vi "Culab Read RF Bin without indicator and warmup.vi"(11 "file path":path=path "E:/TEMP.BIN") -> (3 "exec time":dbl)   [LabVIEW 2020]
uses:
  <vilib>/Ngene/CuLab - GPU Accelerated Toolkit/Toolkit/Low_Level/Tensor_Classes/T_Children/T2D/Controls/T2D_Dims.ctl
  <vilib>/Ngene/CuLab - GPU Accelerated Toolkit/Toolkit/API/Array/Controls/Array_Major.ctl
  <vilib>/Ngene/CuLab - GPU Accelerated Toolkit/Toolkit/Low_Level/Tensor_Classes/T_Children/T1D/T1D_Children/T1D_I16/T1D_I16.lvclass
  C:/Program Files/National Instruments/LabVIEW 2020/vi.lib/Ngene/CuLab - GPU Accelerated Toolkit/Toolkit/Low_Level/Tensor_Classes/T_Children/T1D/T1D.lvclass
  <vilib>/Ngene/CuLab - GPU Accelerated Toolkit/Toolkit/Low_Level/Tensor_Classes/T_Children/T1D/T1D_Children/T1D_CSG/T1D_CSG.lvclass
  <vilib>/Ngene/CuLab - GPU Accelerated Toolkit/Toolkit/Low_Level/Tensor_Classes/T_Children/T1D/T1D_Children/T1D_SGL/Create.vi
  <vilib>/Ngene/CuLab - GPU Accelerated Toolkit/Toolkit/Low_Level/Tensor_Classes/T_Children/T1D/T1D_Children/T1D_I16/Create.vi
  <vilib>/Ngene/CuLab - GPU Accelerated Toolkit/Toolkit/Low_Level/Tensor_Classes/T_Children/T1D/T1D_Children/T1D_CSG/Create.vi
  <vilib>/Ngene/CuLab - GPU Accelerated Toolkit/Toolkit/Low_Level/Tensor_Classes/T_Children/T1D/T1D_Children/T1D_I16/Push.vi
  <vilib>/Ngene/CuLab - GPU Accelerated Toolkit/Toolkit/API/Numeric/Conversion  (API)/SGL/CU_To_SGL_T1D.vi
  <vilib>/Ngene/CuLab - GPU Accelerated Toolkit/Toolkit/API/Numeric/Divide/T1D/CU_DivideC_T1D_SGL.vi
  <vilib>/Ngene/CuLab - GPU Accelerated Toolkit/Toolkit/API/Array/Reshape Array  (API)/CU_Reshape_to_T2D/T1D/CU_Reshape_to_T2D_(T1D_SGL).vi
  <vilib>/Ngene/CuLab - GPU Accelerated Toolkit/Toolkit/API/Array/Index Array Subset/T2D/CU_Index_Array_Subset_T2D_SGL.vi
  <vilib>/Ngene/CuLab - GPU Accelerated Toolkit/Toolkit/API/Numeric/Complex  (API)/Re Im To Complex/T1D/CU_Re_Im_To_Complex_T1D_SGL.vi
  <vilib>/Ngene/CuLab - GPU Accelerated Toolkit/Toolkit/API/Signal Processing/Transforms/CU_FFT/T1D/CU_FFT_T1D_C2C.vi
  <vilib>/Ngene/CuLab - GPU Accelerated Toolkit/Toolkit/API/Array/Array Size/CU_Array_Size_T1D.vi
  <vilib>/Ngene/CuLab - GPU Accelerated Toolkit/Toolkit/API/Numeric/Divide/T1D/CU_DivideC_T1D_CSG.vi
  <vilib>/Ngene/CuLab - GPU Accelerated Toolkit/Toolkit/API/Numeric/Complex  (API)/Complex to Polar/T1D/CU_Complex_to_Polar_T1D_CSG.vi
  <vilib>/Ngene/CuLab - GPU Accelerated Toolkit/Toolkit/API/Elementary/Exponential/Logarithm Base 10/T1D/CU_Logarithm_Base_10_T1D_SGL.vi
  <vilib>/Ngene/CuLab - GPU Accelerated Toolkit/Toolkit/API/Numeric/Multiply/T1D/CU_MultiplyC_T1D_SGL.vi
  <vilib>/Ngene/CuLab - GPU Accelerated Toolkit/Toolkit/API/Numeric/Add/T1D/CU_AddC_T1D_SGL.vi
  <vilib>/Ngene/CuLab - GPU Accelerated Toolkit/Toolkit/Low_Level/Tensor_Classes/T_Children/T1D/T1D_Children/T1D_SGL/Pull.vi
  <vilib>/Ngene/CuLab - GPU Accelerated Toolkit/Toolkit/CuLab.lvlib
  <vilib>/Ngene/CuLab - GPU Accelerated Toolkit/Toolkit/Low_Level/Tensor_Classes/T_Children/T1D/T1D_Children/T1D_SGL/T1D_SGL.lvclass
  <vilib>/Ngene/CuLab - GPU Accelerated Toolkit/Toolkit/Low_Level/Tensor_Classes/T_Children/T2D/T2D_Children/T2D_CDB/T2D_CDB.lvclass
  C:/Program Files/National Instruments/LabVIEW 2020/vi.lib/Ngene/CuLab - GPU Accelerated Toolkit/Toolkit/Low_Level/Tensor_Classes/Tensor.lvclass
  C:/Program Files/National Instruments/LabVIEW 2020/vi.lib/Ngene/CuLab - GPU Accelerated Toolkit/Toolkit/Low_Level/Tensor_Classes/T_Children/T1D/T1D_Children/T1D_I16/T1D_I16.lvclass
  C:/Program Files/National Instruments/LabVIEW 2020/vi.lib/Ngene/CuLab - GPU Accelerated Toolkit/Toolkit/Low_Level/Tensor_Classes/T_Children/T1D/T1D_Children/T1D_CSG/T1D_CSG.lvclass
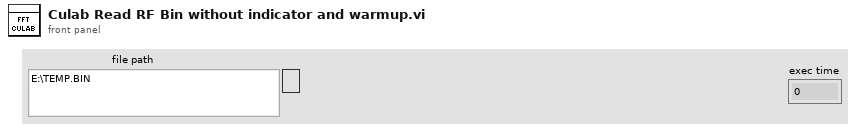
[diagram p1: front panel]
types:
  T1 = enum16{"open", "replace", "create", "open or create", "replace or create", "replace or create with confirmation"}
  T2 = typedef "CuLab.lvlib/T2D_Dims.ctl" = cluster{"H":i32, "W":i32}
  T3 = enum16{"big-endian, network order", "native, host order", "little-endian"}
  T4 = typedef "CuLab.lvlib/Array_Major.ctl" = enum16{"Row", "Column"}
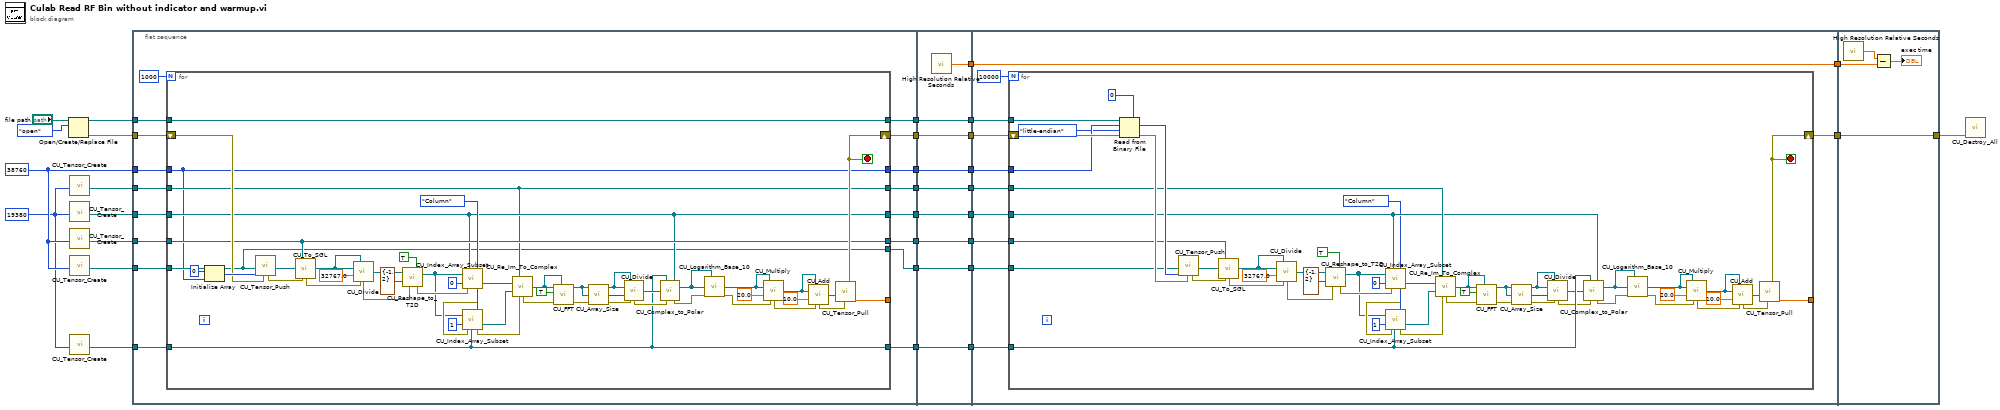
[diagram p0: block diagram]
diagram:
  w21 = 19380 ("count (1)")
  w24 = 38760 ("count (1)")
  n1 = Open/Create/Replace File(file path (use dialog)="file path", operation (0:open)=T1."open") -> (refnum out=w29:refnum<file>, error out=w9:errorcluster)  [unwired: 4 in, 1 out]
  n2 = call-poly <vilib>:"CU_Tensor_Create.vi"("Length"=w21) -> ("T1D_CSG out"=w26:refnum<class "T1D_CSG.lvclass">)  [unwired: 9 in, 1 out]
  n3 = call-poly <vilib>:"CU_Tensor_Create.vi"("Length"=w21) -> ("T1D_SGL out"=w25:refnum<class "T1D_SGL.lvclass">)  [unwired: 9 in, 1 out]
  n4 = call-poly <vilib>:"CU_Tensor_Create.vi"("Length"=w24) -> ("T1D_SGL out"=w27:refnum<class "T1D_SGL.lvclass">)  [unwired: 9 in, 1 out]
  n5 = call-poly <vilib>:"CU_Tensor_Create.vi"("Length"=w24) -> ("T1D_I16 out"=w28:refnum<class "T1D_I16.lvclass">)  [unwired: 9 in, 1 out]
  n6 = call-poly <vilib>:"CU_Tensor_Create.vi"("Length"=w21) -> ("T1D_SGL out"=w23:refnum<class "T1D_SGL.lvclass">)  [unwired: 9 in, 1 out]
  n7 = flat-sequence {
    tunnel: w9 -> [w47]
    tunnel: w23 -> [w43]
    tunnel: w24 -> [w45]
    tunnel: w25 -> [w41]
    tunnel: w26 -> [w40]
    tunnel: w27 -> [w42]
    tunnel: w28 -> [w44]
    tunnel: w29 -> [w46]
    tunnel: [w36] -> w8
    tunnel: [w39] -> w7
    tunnel: [w38] -> w6
    tunnel: [w37] -> w5
    tunnel: [w35] -> w4
    tunnel: [w34] -> w3
    tunnel: [w33] -> w2
    tunnel: [w32] -> w1
    tunnel: [w105] -> w20
    tunnel: [w104] -> w19
    tunnel: [w103] -> w18
    tunnel: [w102] -> w17
    tunnel: [w101] -> w16
    tunnel: [w100] -> w15
    tunnel: [w99] -> w14
    tunnel: [w98] -> w12
    tunnel: [w97] -> w10
    tunnel: w8 -> [w104]
    tunnel: w7 -> [w103]
    tunnel: w6 -> [w101]
    tunnel: w5 -> [w102]
    tunnel: w4 -> [w99]
    tunnel: w3 -> [w97]
    tunnel: w2 -> [w105]
    tunnel: w1 -> [w100]
    tunnel: w20 -> [w115]
    tunnel: w19 -> [w114]
    tunnel: w18 -> [w113]
    tunnel: w17 -> [w112]
    tunnel: w16 -> [w111]
    tunnel: w15 -> [w110]
    tunnel: w14 -> [w109]
    tunnel: [w108] -> w13
    tunnel: w12 -> [w107]
    tunnel: [w107] -> w11
    tunnel: w10 -> [w106]
    tunnel: [w170] -> w22
    tunnel: w13 -> [w170]
    tunnel: w11 -> [w168]
    frame #0 {
      n8 = for {
        N: 1000 -> [_]
        shift-right: [w94] -> w34
        shift-left: w47 -> [w56]
        tunnel: w46 -> [w50]
        tunnel: w44 -> [w52]
        tunnel: w45 -> [w49]
        tunnel: w42 -> [w55]
        tunnel: w40 -> [w53]
        tunnel: w41 -> [w54]
        tunnel: w43 -> [w51]
        tunnel: [w59] -> _
        tunnel: [w55] -> w39
        tunnel: [w54] -> w38
        tunnel: [w53] -> w37
        tunnel: [w52] -> w36
        tunnel: [w51] -> w35
        tunnel: [w50] -> w33
        tunnel: [w49] -> w32
        stop <- w94 stop-if-true
        w87 = Array_Major."Column" ("Row/Column Selector")
        n9 = Initialize Array(i16 0 ("element"), w49) -> (w57:i16[])
        n10 = call-poly <vilib>:"CU_Tensor_Push.vi"("error in (no error)"=w56, "T1D_I16_Data"=w57, "T1D_I16 in"=w52) -> ("T1D_I16 out"=w82:refnum<class "T1D_I16.lvclass">, "error out"=w74:errorcluster)  [unwired: 7 in]
        n11 = call-poly <vilib>:"CU_To_SGL.vi"("Dest in"=w55, "Tensor in"=w82, "error in (no error)"=w74) -> ("Dest out"=w81:refnum<class "T1D_SGL.lvclass">, "error out"=w73:errorcluster)  [unwired: 11 in]
        n12 = call-poly <vilib>:"CU_Divide.vi"("Dest in"=w81, "x"=w81, "y"=sgl 32767.0 ("Numeric"), "error in (no error)"=w73) -> ("Dest out"=w92:refnum<class "T1D_SGL.lvclass">, "error out"=w72:errorcluster)  [unwired: 10 in]
        n13 = call-poly <vilib>:"CU_Reshape_to_T2D.vi"("InPlace?(F)"=TRUE, "Tensor in"=w92, "Target Dim"=T2 {"H"=-1, "W"=2}, "error in (no error)"=w72) -> ("Dest out"=w62:refnum<class "T2D_SGL.lvclass">, "error out"=w71:errorcluster)  [unwired: 10 in]
        n14 = call-poly <vilib>:"CU_Index_Array_Subset.vi"("Tensor in"=w62, "Index"=0, "error in (no error)"=w71, "Dest in"=w54, "Row/Column Selector"=w87) -> ("error out"=w70:errorcluster, "Sub Tensor"=w61:refnum<class "T1D_SGL.lvclass">)  [unwired: 13 in]
        n15 = call-poly <vilib>:"CU_Index_Array_Subset.vi"("Tensor in"=w62, "Index"=1, "error in (no error)"=w70, "Dest in"=w51, "Row/Column Selector"=w87) -> ("error out"=w69:errorcluster, "Sub Tensor"=w60:refnum<class "T1D_SGL.lvclass">)  [unwired: 13 in]
        n16 = call-poly <vilib>:"CU_Re_Im_To_Complex.vi"("Dest in"=w53, "x"=w61, "y"=w60, "error in (no error)"=w69) -> ("Dest out"=w76:refnum<class "T1D_CSG.lvclass">, "error out"=w68:errorcluster)  [unwired: 10 in]
        n17 = call-poly <vilib>:"CU_FFT.vi"("FFT {X} dest"=w76, "error in"=w68, "shift?"=TRUE, "X"=w76) -> ("error out"=w67:errorcluster, "FFT {X}"=w77:refnum<class "T1D_CSG.lvclass">)  [unwired: 6 in]
        n18 = call-poly <vilib>:"CU_Array_Size.vi"("Tensor"=w77) -> ("size"=w86:i32)  [unwired: 14 in]
        n19 = call-poly <vilib>:"CU_Divide.vi"("Dest in"=w77, "x"=w77, "y"=w86, "error in (no error)"=w67) -> ("Dest out"=w85:refnum<class "T1D_CSG.lvclass">, "error out"=w66:errorcluster)  [unwired: 10 in]
        n20 = call-poly <vilib>:"CU_Complex_to_Polar.vi"("r Dest in"=w51, "theta Dest in"=w54, "r * e^(i*theta)"=w85, "error in (no error)"=w66) -> ("r out"=w78:refnum<class "T1D_SGL.lvclass">, "error out"=w65:errorcluster)  [unwired: 9 in, 1 out]
        n21 = call-poly <vilib>:"CU_Logarithm_Base_10.vi"("Dest in"=w78, "x"=w78, "error in (no error)"=w65) -> ("log(x)"=w79:refnum<class "T1D_SGL.lvclass">, "error out"=w64:errorcluster)  [unwired: 11 in]
        n22 = call-poly <vilib>:"CU_Multiply.vi"("Dest in"=w79, "x"=w79, "y"=sgl 20.0 ("Numeric"), "error in (no error)"=w64) -> ("Dest out"=w80:refnum<class "T1D_SGL.lvclass">, "error out"=w63:errorcluster)  [unwired: 10 in]
        n23 = call-poly <vilib>:"CU_Add.vi"("Dest in"=w80, "x"=w80, "y"=sgl 10.0 ("Numeric"), "error in (no error)"=w63) -> ("Dest out"=w96:refnum<class "T1D_SGL.lvclass">, "error out"=w95:errorcluster)  [unwired: 10 in]
        n24 = call-poly <vilib>:"CU_Tensor_Pull.vi"("error in (no error)"=w95, "T1D_SGL in"=w96) -> ("Dest out"=w59:sgl[], "error out"=w94:errorcluster)  [unwired: 7 in, 1 out]
      }
    }
    frame #1 {
      n25 = call <vilib>:"High Resolution Relative Seconds.vi"() -> ("relative seconds"=w98:dbl)
    }
    frame #2 {
      n26 = for {
        N: 10000 -> [_]
        shift-right: [w154] -> w108
        shift-left: w106 -> [w166]
        tunnel: w115 -> [w165]
        tunnel: w114 -> [w161]
        tunnel: w110 -> [w160]
        tunnel: w113 -> [w159]
        tunnel: w112 -> [w158]
        tunnel: w111 -> [w157]
        tunnel: w109 -> [w156]
        tunnel: [w117] -> _
        stop <- w154 stop-if-true
        w145 = Array_Major."Column" ("Row/Column Selector")
        n27 = Read from Binary File(5:i16 0 ("Numeric"), 8:w166, 9:T3."little-endian" ("byte order (0:big-endian, network order)"), 10:w160, 11:w165) -> (0:w163:errorcluster, 2:w164:i16[])  [unwired: 1 in, 2 out]
        n28 = call-poly <vilib>:"CU_Tensor_Push.vi"("error in (no error)"=w163, "T1D_I16_Data"=w164, "T1D_I16 in"=w161) -> ("T1D_I16 out"=w140:refnum<class "T1D_I16.lvclass">, "error out"=w132:errorcluster)  [unwired: 7 in]
        n29 = call-poly <vilib>:"CU_To_SGL.vi"("Dest in"=w159, "Tensor in"=w140, "error in (no error)"=w132) -> ("Dest out"=w139:refnum<class "T1D_SGL.lvclass">, "error out"=w131:errorcluster)  [unwired: 11 in]
        n30 = call-poly <vilib>:"CU_Divide.vi"("Dest in"=w139, "x"=w139, "y"=sgl 32767.0 ("Numeric"), "error in (no error)"=w131) -> ("Dest out"=w150:refnum<class "T1D_SGL.lvclass">, "error out"=w130:errorcluster)  [unwired: 10 in]
        n31 = call-poly <vilib>:"CU_Reshape_to_T2D.vi"("InPlace?(F)"=TRUE, "Tensor in"=w150, "Target Dim"=T2 {"H"=-1, "W"=2}, "error in (no error)"=w130) -> ("Dest out"=w120:refnum<class "T2D_SGL.lvclass">, "error out"=w129:errorcluster)  [unwired: 10 in]
        n32 = call-poly <vilib>:"CU_Index_Array_Subset.vi"("Tensor in"=w120, "Index"=0, "error in (no error)"=w129, "Dest in"=w157, "Row/Column Selector"=w145) -> ("error out"=w128:errorcluster, "Sub Tensor"=w119:refnum<class "T1D_SGL.lvclass">)  [unwired: 13 in]
        n33 = call-poly <vilib>:"CU_Index_Array_Subset.vi"("Tensor in"=w120, "Index"=1, "error in (no error)"=w128, "Dest in"=w156, "Row/Column Selector"=w145) -> ("error out"=w127:errorcluster, "Sub Tensor"=w118:refnum<class "T1D_SGL.lvclass">)  [unwired: 13 in]
        n34 = call-poly <vilib>:"CU_Re_Im_To_Complex.vi"("Dest in"=w158, "x"=w119, "y"=w118, "error in (no error)"=w127) -> ("Dest out"=w134:refnum<class "T1D_CSG.lvclass">, "error out"=w126:errorcluster)  [unwired: 10 in]
        n35 = call-poly <vilib>:"CU_FFT.vi"("FFT {X} dest"=w134, "error in"=w126, "shift?"=TRUE, "X"=w134) -> ("error out"=w125:errorcluster, "FFT {X}"=w135:refnum<class "T1D_CSG.lvclass">)  [unwired: 6 in]
        n36 = call-poly <vilib>:"CU_Array_Size.vi"("Tensor"=w135) -> ("size"=w144:i32)  [unwired: 14 in]
        n37 = call-poly <vilib>:"CU_Divide.vi"("Dest in"=w135, "x"=w135, "y"=w144, "error in (no error)"=w125) -> ("Dest out"=w143:refnum<class "T1D_CSG.lvclass">, "error out"=w124:errorcluster)  [unwired: 10 in]
        n38 = call-poly <vilib>:"CU_Complex_to_Polar.vi"("r Dest in"=w156, "theta Dest in"=w157, "r * e^(i*theta)"=w143, "error in (no error)"=w124) -> ("r out"=w136:refnum<class "T1D_SGL.lvclass">, "error out"=w123:errorcluster)  [unwired: 9 in, 1 out]
        n39 = call-poly <vilib>:"CU_Logarithm_Base_10.vi"("Dest in"=w136, "x"=w136, "error in (no error)"=w123) -> ("log(x)"=w137:refnum<class "T1D_SGL.lvclass">, "error out"=w122:errorcluster)  [unwired: 11 in]
        n40 = call-poly <vilib>:"CU_Multiply.vi"("Dest in"=w137, "x"=w137, "y"=sgl 20.0 ("Numeric"), "error in (no error)"=w122) -> ("Dest out"=w138:refnum<class "T1D_SGL.lvclass">, "error out"=w121:errorcluster)  [unwired: 10 in]
        n41 = call-poly <vilib>:"CU_Add.vi"("Dest in"=w138, "x"=w138, "y"=sgl 10.0 ("Numeric"), "error in (no error)"=w121) -> ("Dest out"=w162:refnum<class "T1D_SGL.lvclass">, "error out"=w155:errorcluster)  [unwired: 10 in]
        n42 = call-poly <vilib>:"CU_Tensor_Pull.vi"("error in (no error)"=w155, "T1D_SGL in"=w162) -> ("Dest out"=w117:sgl[], "error out"=w154:errorcluster)  [unwired: 7 in, 1 out]
      }
    }
    frame #3 {
      n43 = call <vilib>:"High Resolution Relative Seconds.vi"() -> ("relative seconds"=w169:dbl)
      n44 = Subtract(x=w169, y=w168) -> (x-y=→"exec time":dbl)
    }
  }
  n45 = call <vilib>:"CU_Destroy_All.vi"("error in"=w22) -> ()  [unwired: 10 in, 1 out]
